vi "WaitMultiple.vi"(7 "wait option?":i32(ring) items=["MoveDone", "InPosition"], 8 "error in (no error)":errorcluster, 9 "timeout? (msec)":i32=-1, 10 "axis names":string[](array[string]), 11 "controller in":refnum<k24>) -> (0 "error out":errorcluster, 2 "completed":bool, 3 "controller out":refnum<k24>)   [LabVIEW 2021, in "Aerotech.lvlib"]
uses:
  Users/hep/Aerotech.lvlib
  C:/Program Files (x86)/Aerotech/A3200/LabVIEW/2010/Bin/Aerotech.A3200.LabVIEW.dll
  Bin/Aerotech.A3200.LabVIEW.dll
  C:/Program Files (x86)/Aerotech/A3200/LabVIEW/2010/Bin/Aerotech.A3200.dll
  Bin/Aerotech.A3200.dll
panel:
  in  "taskId":i32(ring) items=["TLibrary", "T01", "T02", "T03", "T04", "T05", "T06", "T07", "T08", "T09", "T10", "T11", "T12", "T13", "T14", "T15", "T16", "T17", "T18", "T19", "T20", "T21", "T22", "T23", "T24", "T25", "T26", "T27", "T28", "T29", "T30", "T31"]
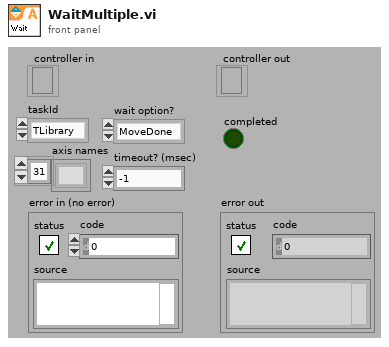
[diagram p1: front panel]
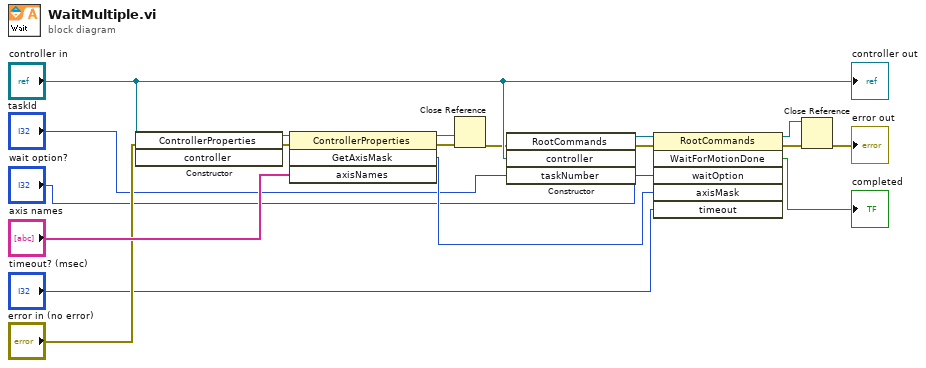
[diagram p0: block diagram]
diagram:
  n1 = constructor class="ControllerProperties"(error in="error in (no error)", "controller"="controller in") -> (reference out=w16:refnum<k24>, error out=w15:errorcluster)  [unwired: 2 in, 2 out]
  n2 = invoke class="ControllerProperties" method="GetAxisMask"(reference=w16, error in=w15, "axisNames"="axis names") -> (reference out=w13:refnum<k24>, error out=w14:errorcluster, "GetAxisMask"=w9:i32)  [unwired: 1 in, 1 out]
  n3 = Close Reference(reference=w13, error in (no error)=w14) -> (error out=w4:errorcluster)
  n4 = constructor class="RootCommands"(error in=w4, "controller"="controller in", "taskNumber"="taskId") -> (reference out=w3:refnum<k24>, error out=w2:errorcluster)  [unwired: 2 in, 3 out]
  n5 = invoke class="RootCommands" method="WaitForMotionDone"(reference=w3, error in=w2, "waitOption"="wait option?", "axisMask"=w9, "timeout"="timeout? (msec)") -> (reference out=w17:refnum<k24>, error out=w18:errorcluster, "WaitForMotionDone"=→"completed":bool)  [unwired: 1 in, 3 out]
  n6 = Close Reference(reference=w17, error in (no error)=w18) -> (error out=→"error out":errorcluster)
  "controller out" <- "controller in"
